vi "conversational read pending signals.vi"(0 "Serial Port":refnum<visa-resource-name>, 1 "data points":u8=5, 2 "signals":enum16{"signal 1", "signals 1 and 2"}(ring)=enum."signals 1 and 2", 5 "Max time (ms)":u32=2000, 9 "signal 1 in":dbl[](array[numeric]) format="%.2f", 11 "signal 2 in":dbl[](array[numeric]) format="%.2f", 12 "i":i32) -> (4 "Serial Port":refnum<visa-resource-name>, 8 "run done":bool, 10 "signal 1 out":dbl[](array[numeric]) format="%.2f", 14 "last data":dbl[](array[numeric]) format="%.2f", 15 "signal 2 out":dbl[](array[numeric]) format="%.2f")   [LabVIEW 2012]
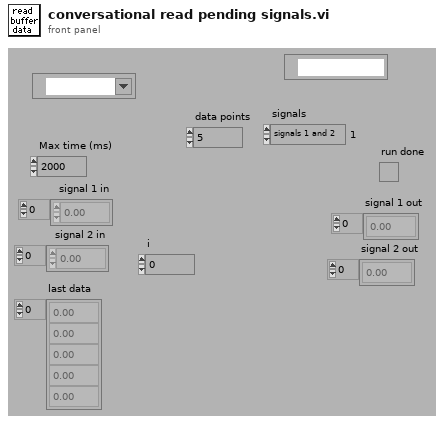
[diagram p1: front panel]
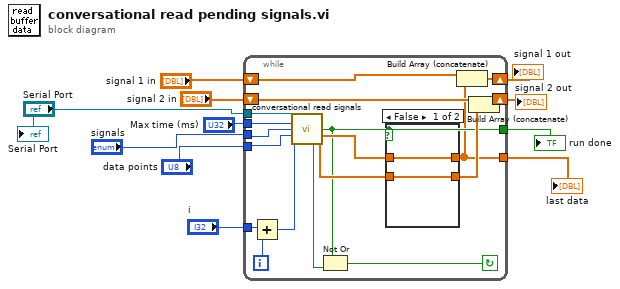
[diagram p0: block diagram]
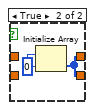
[diagram p2: hidden frame]
diagram:
  n1 = while {
    tunnel: [w12] -> w1
    tunnel: [w14] -> w3
    tunnel: "i" -> [w17]
    tunnel: "Max time (ms)" -> [w20]
    tunnel: "data points" -> [w18]
    tunnel: "signals" -> [w19]
    tunnel: "Serial Port" -> [w24]
    shift-left: "signal 2 in" -> [w29]
    shift-right: [w26] -> w11
    shift-left: "signal 1 in" -> [w28]
    shift-right: [w27] -> w10
    i -> [w16]
    stop <- w15 continue-if-true
    n2 = Add(x=w17, y=w16) -> (x+y=w13:i32)
    n3 = call "conversational read signals.vi"("Serial Port"=w24, "Max time (ms)"=w20, "signals"=w19, "data points"=w18, "i"=w13) -> ("run done"=w14:bool, "signal 1"=w23:dbl[], "emptied buffer"=w21:bool, "signal 2"=w22:dbl[])  [unwired: 4 in, 3 out]
    n4 = Not Or(1:w21, 2:w14) -> (0:w15:bool)
    n5 = case shown="False" w14 {
      tunnel: w23 -> [w31 _]
      tunnel: [w31 w32] -> w12
      tunnel: [w30 w32] -> w25
      tunnel: w22 -> [w30 _]
      frame False {
      }
      frame True {
        w33 = 0
        n6 = Initialize Array(w33, w33) -> (w32:i32[])
      }
    }
    n7 = Build Array (concatenate)(w28, w12) -> (w27:dbl[])
    n8 = Build Array (concatenate)(w29, w25) -> (w26:dbl[])
  }
  "signal 1 out" <- w10
  "signal 2 out" <- w11
  "run done" <- w3
  "last data" <- w1
  "Serial Port" <- "Serial Port"
